vi "Pixel_LIDAR_Run_old.vi"(1 "Noise (0.1 to 1)":dbl, 4 "Initial\nSonarRay\nArray":i32[](array[numeric]), 5 "error in (no error)":errorcluster, 6 "SonarRange":dbl=20.0 min=20.0 max=300.0, 7 "NumberOfBeams":i32=1 min=1 max=360 step=1, 8 "SubPosition":cluster{"xsub":dbl, "ysub":dbl, "heading":dbl}, 9 "MDF Image In":T1) -> (0 "error out":errorcluster, 2 "Collision\nWarning":bool, 3 "Sonar Data (r:pixel b:degrees)":cluster{"Range":dbl, "Bearing":dbl}[](array[cluster]))   [LabVIEW 2010]
doc: "This SubVI takes the TunaSub's current position and heading and MDF and calculates the sonar range to shore along a set of evenly spaced sonar rays over a fixed sensor range.\nIt looks for the pixel color change from blue (255) to anything to calculate range."
uses:
  <vilib>/vision/Image Controls.llb/IMAQ Image.ctl
  <vilib>/vision/NI_Vision_Development_Module.lvlib
panel:
  # "This SubVI takes TunaSub's current position and orientaton and MDF and calculates the sonar range to shore along a set of evenly spaced sonar beams (NumberOfBeams) over a fixed sensor range (SonarRange)"
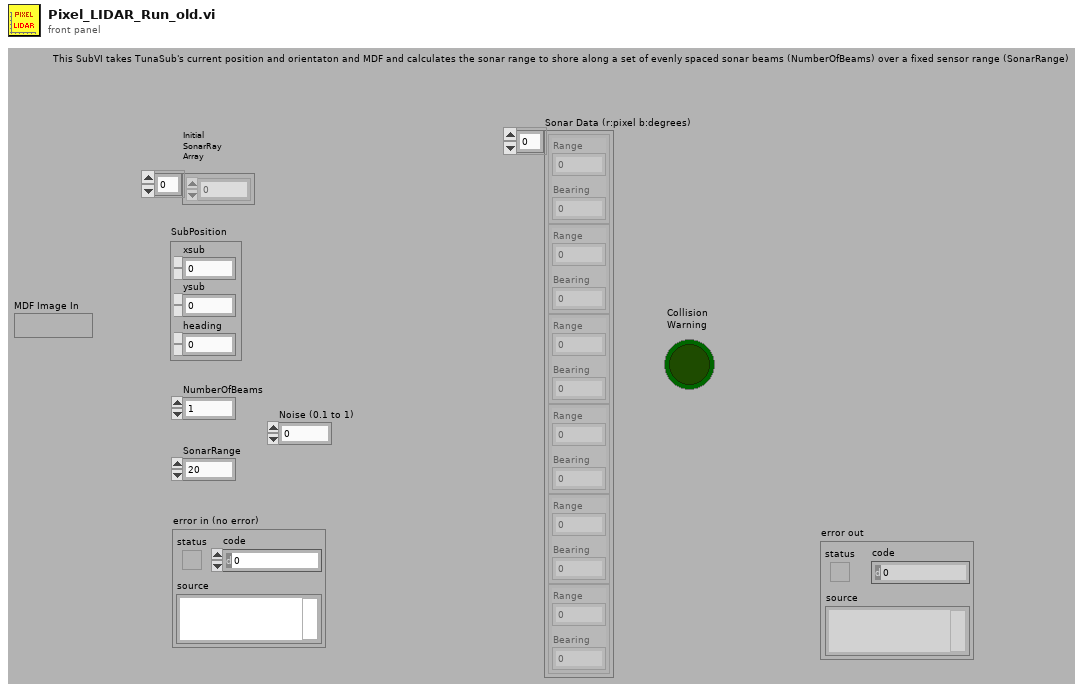
[diagram p1: front panel]
types:
  T1 = typedef "IMAQ Image.ctl" = refnum<image>
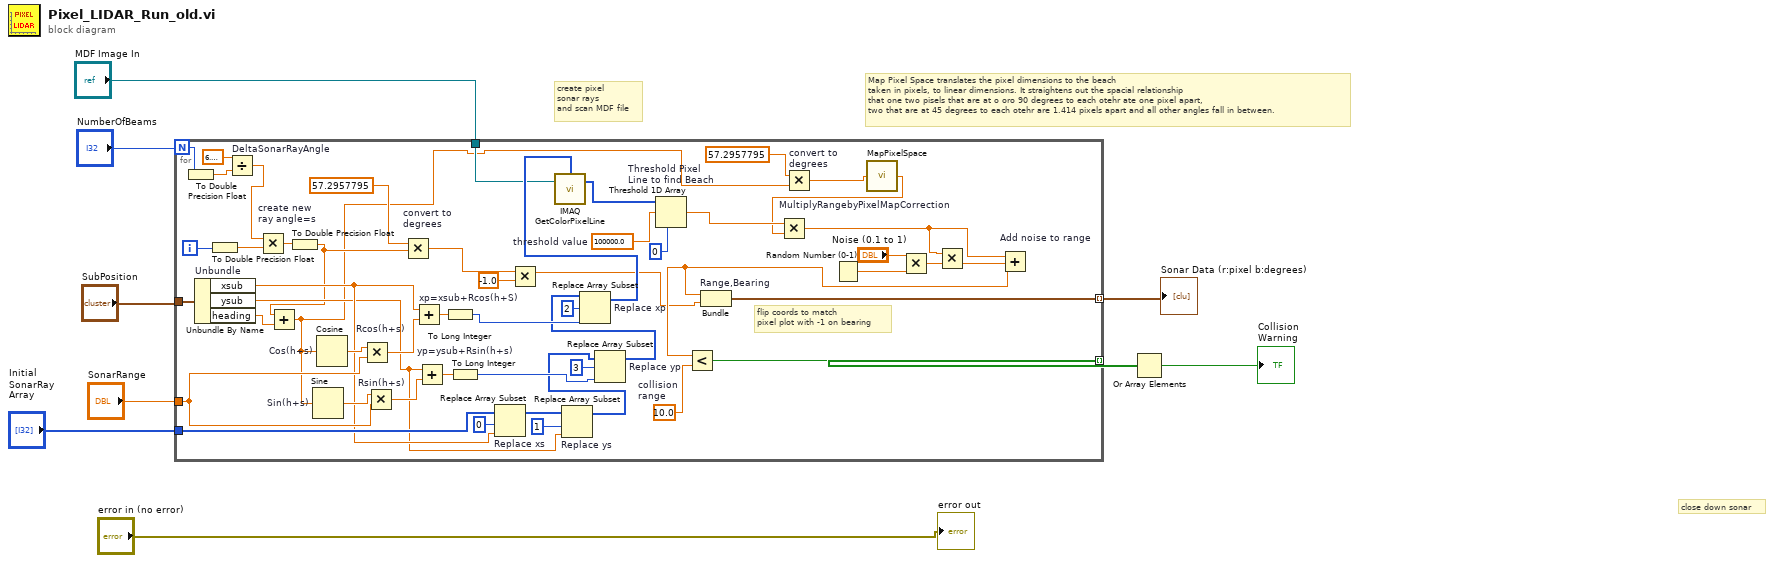
[diagram p0: block diagram]
diagram:
  # "Map Pixel Space translates the pixel dimensions to the beach\ntaken in pixels, to linear dimensions. It straightens out the spacial relationship \nthat one two pisels that are at o oro 90 degrees to each otehr ate one pixel apart,\ntwo that are at 45 degrees to each otehr are 1.414 pixels apart and all other angles fall in between."
  # "create pixel \nsonar rays\nand scan MDF file"
  # "close down sonar"
  n1 = for {
    N: "NumberOfBeams" -> [w39]
    tunnel: "SonarRange" -> [w58]
    tunnel: "SubPosition" -> [w61]
    tunnel: "MDF Image In" -> [w33]
    tunnel: "Initial\nSonarRay\nArray" -> [w48]
    tunnel: [w30] -> w3 mode=indexing
    tunnel: [w27] -> w2 mode=indexing
    i -> [w35]
    w28 = 10.0  # collision range
    w32 = 100000.0  # threshold value
    # "flip coords to match\npixel plot with -1 on bearing"
    n2 = To Double Precision Float(number=w39) -> (double precision float=w37:dbl)
    n3 = Unbundle By Name "Unbundle"(w61) -> ("xsub"=w43:dbl, "ysub"=w42:dbl, "heading"=w22:dbl)
    n4 = To Double Precision Float(number=w35) -> (double precision float=w36:dbl)
    n5 = Divide "DeltaSonarRayAngle"(x=6.283185307179586, y=w37) -> (x/y=w38:dbl)
    n6 = Multiply "create new \nray angle=s"(x=w38, y=w36) -> (x*y=w41:dbl)
    n7 = To Double Precision Float(number=w41) -> (double precision float=w21:dbl)
    n8 = Add(x=w21, y=w22) -> (x+y=w18:dbl)
    n9 = Sine "Sin(h+s)"(x=w18) -> (sin(x)=w56:dbl)
    n10 = Cosine "Cos(h+s)"(x=w18) -> (cos(x)=w57:dbl)
    n11 = Multiply "Rcos(h+s)"(x=w57, y=w58) -> (x*y=w60:dbl)
    n12 = Multiply "Rsin(h+s)"(x=w56, y=w58) -> (x*y=w59:dbl)
    n13 = Multiply "convert to\ndegrees"(x=57.2957795 ("y"), y=w21) -> (x*y=w23:dbl)
    n14 = Add "xp=xsub+Rcos(h+S)"(x=w43, y=w60) -> (x+y=w52:dbl)
    n15 = Add "yp=ysub+Rsin(h+s)"(x=w42, y=w59) -> (x+y=w53:dbl)
    n16 = To Long Integer(number=w52) -> (32bit integer=w51:i32)
    n17 = To Long Integer(number=w53) -> (32bit integer=w50:i32)
    n18 = Replace Array Subset "Replace xs"(array=w48, new element=w43, index=0) -> (w47:i32[])
    n19 = Multiply(x=w23, y=-1.0) -> (x*y=w11:dbl)
    n20 = Replace Array Subset "Replace ys"(array=w47, new element=w42, index=1) -> (w46:i32[])
    n21 = Replace Array Subset "Replace yp"(array=w46, new element=w50, index=3) -> (w49:i32[])
    n22 = Replace Array Subset "Replace xp"(array=w49, new element=w51, index=2) -> (w34:i32[])
    n23 = call "IMAQ GetColorPixelLine"("Line Coordinates"=w34, "Image"=w33) -> ("Pixels Line (U32)"=w29:u32[])  [unwired: 2 in, 2 out]
    n24 = Threshold 1D Array "Threshold Pixel\nLine to find Beach"(1:0 ("start index (0)"), 2:w32, 3:w29) -> (0:w25:dbl)
    n25 = Multiply "convert to\ndegrees"(x=57.2957795 ("y"), y=w18) -> (x*y=w20:dbl)
    n26 = Random Number (0-1)() -> (number: 0 to 1=w17:dbl)
    n27 = call "MapPixelSpace.vi"("angle (deg)"=w20) -> ("spacemapout"=w24:dbl)
    n28 = Multiply "MultiplyRangebyPixelMapCorrection"(x=w25, y=w24) -> (x*y=w12:dbl)
    n29 = Multiply ("add noise in")(x="Noise (0.1 to 1)", y=w17) -> (x*y=w15:dbl)
    n30 = Multiply(x=w12, y=w15) -> (x*y=w13:dbl)
    n31 = Add "Add noise to range"(x=w12, y=w13) -> (x+y=w14:dbl)
    n32 = Less?(x=w14, y=w28) -> (x < y?=w27:bool)
    n33 = Bundle "Range,Bearing"(w14, w11) -> (w30:cluster{dbl, dbl})  [unwired: 1 in]
  }
  "Sonar Data (r:pixel b:degrees)" <- w3
  n34 = Or Array Elements(Boolean array=w2) -> (logical OR=→"Collision\nWarning":bool)
  "error out" <- "error in (no error)"
